vi "Connect.vi"(8 "error in (no error)":errorcluster, 10 "Connect?":bool, 11 "Reload-pro in":refnum<class "Reload-pro.lvclass">) -> (0 "error out":errorcluster, 3 "Reload-pro out":refnum<class "Reload-pro.lvclass">)   [LabVIEW 2013, in "Reload-pro.lvclass"]
uses:
  Reload-pro.lvclass
  Reload-pro.lvclass/Reload-pro.ctl
  <vilib>/Instr/_visa.llb/VISA Configure Serial Port (Instr).vi
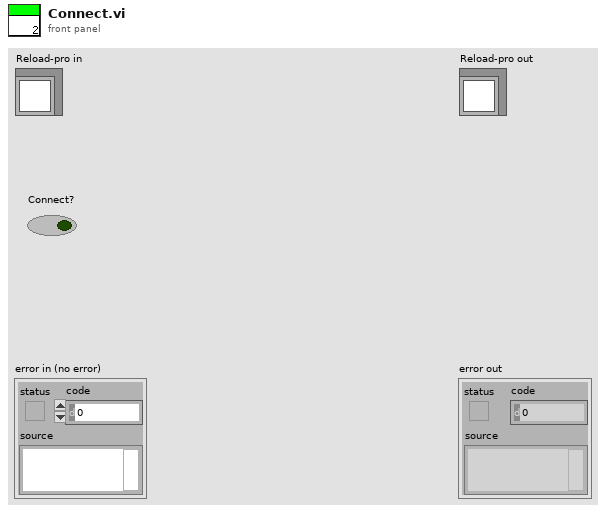
[diagram p1: front panel]
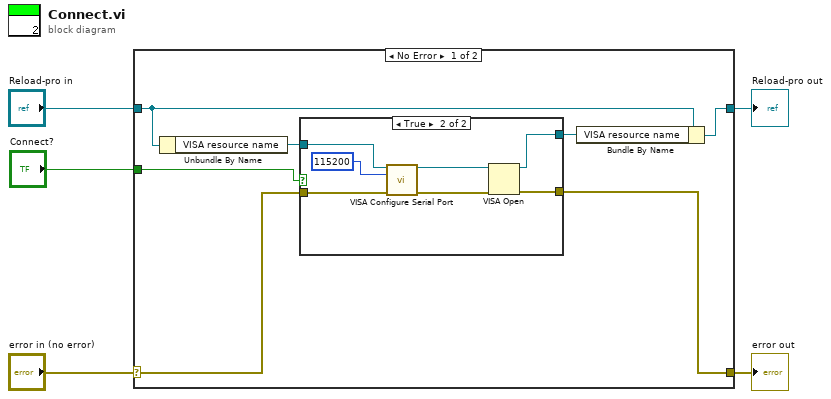
[diagram p0: block diagram]
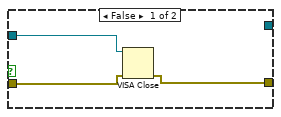
[diagram p2: hidden frame]
diagram:
  n1 = case shown="No Error" "error in (no error)" {
    selector: "error in (no error)" -> [w8 w24]
    tunnel: [w7 w24] -> w4
    tunnel: [w12 w23] -> w2
    tunnel: "Reload-pro in" -> [w11 w23]
    tunnel: "Connect?" -> [w6 _]
    frame No Error {
      n2 = Unbundle By Name(w11) -> ("VISA resource name"=w9:refnum<visa-resource-name>)
      n3 = case shown="True" w6 {
        tunnel: [_ w22] -> w10
        tunnel: w9 -> [w15 w21]
        tunnel: w8 -> [w14 w17]
        tunnel: [w13 w16] -> w7
        frame False {
          n4 = VISA Close(VISA resource name=w15, error in (no error)=w14) -> (error out=w13:errorcluster)
        }
        frame True {
          n5 = call-poly "VISA Configure Serial Port"("VISA resource name"=w21, "baud rate (9600)"=u32 115200, "error in (no error)"=w17) -> ("VISA resource name out"=w20:refnum<visa-resource-name>, "error out"=w18:errorcluster)  [unwired: 11 in]
          n6 = VISA Open(error in (no error)=w18, VISA resource name=w20) -> (VISA resource name=w22:refnum<visa-resource-name>, error out=w16:errorcluster)  [unwired: 3 in]
        }
      }
      n7 = Bundle By Name(cluster=w11, "VISA resource name"=w10) -> (w12:refnum<class "Reload-pro.lvclass">)
    }
    frame Error {
    }
  }
  "error out" <- w4
  "Reload-pro out" <- w2
